vi "square_brackets_beside_vertical_bar_solution.vi"(8 "error in (no error)":errorcluster, 11 "Instrument Command In":string) -> (0 "error out":errorcluster, 3 "Instrument Command Out":string)   [LabVIEW 2018]
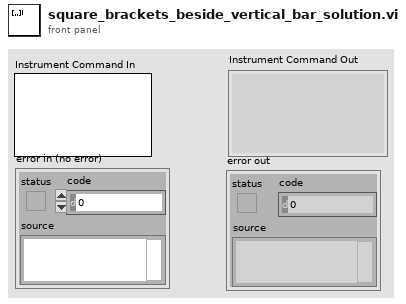
[diagram p1: front panel]
types:
  T1 = cluster{"Start Sting":string, "End String":string}
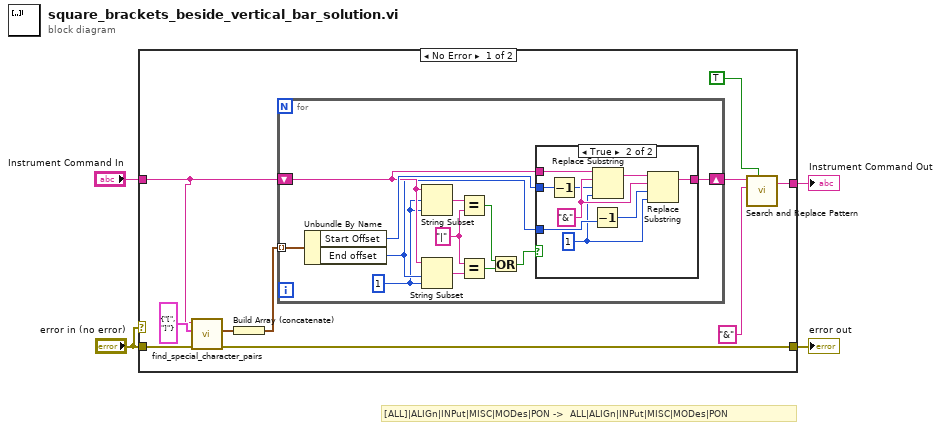
[diagram p0: block diagram]
diagram:
  # "[ALL]|ALIGn|INPut|MISC|MODes|PON ->  ALL|ALIGn|INPut|MISC|MODes|PON"
  n1 = case shown="No Error" "error in (no error)" {
    selector: "error in (no error)" -> [_ w38]
    tunnel: "Instrument Command In" -> [w5 w37]
    tunnel: "error in (no error)" -> [w9 _]
    tunnel: [w8 w38] -> w3
    tunnel: [w6 w37] -> w2
    frame No Error {
      n2 = call "find_special_character_pairs.vi"("error in (no error)"=w9, "String Pair"=T1 {"Start Sting"="[", "End String"="]"}, "Command String"=w5) -> ("error out"=w8:errorcluster, "Pair Offset"=w11:cluster{"Start Offset":i32, "End offset":i32}[])  [unwired: 7 out]
      n3 = Build Array (concatenate)(w11) -> (w10:cluster{"Start Offset":i32, "End offset":i32}[])
      n4 = for {
        shift-right: [w18] -> w13
        shift-left: w5 -> [w19]
        tunnel: w10 -> [w15] mode=indexing
        w24 = "|"
        w16 = 1
        n5 = Unbundle By Name(w15) -> ("Start Offset"=w20:i32, "End offset"=w17:i32)
        n6 = String Subset(string=w19, offset (0)=w16, length (rest)=w16) -> (substring=w26:string)
        n7 = String Subset(string=w19, offset (0)=w17, length (rest)=w16) -> (substring=w25:string)
        n8 = Equal?(x=w26, y=w24) -> (x = y?=w23:bool)
        n9 = Equal?(x=w24, y=w25) -> (x = y?=w22:bool)
        n10 = Or(x=w23, y=w22) -> (x .or. y?=w21:bool)
        n11 = case shown="True" w21 {
          tunnel: w20 -> [_ w36]
          tunnel: w19 -> [w27 w35]
          tunnel: w17 -> [_ w32]
          tunnel: [w27 w30] -> w18
          frame False {
          }
          frame True {
            w33 = "&" ("substring (\"\")")
            w31 = 1 ("length (len. of substring)")
            n12 = Decrement(x=w36) -> (x-1=w28:i32)
            n13 = Decrement(x=w32) -> (x-1=w29:i32)
            n14 = Replace Substring(2:w31, 3:w28, 4:w33, 5:w35) -> (1:w34:string)  [unwired: 1 out]
            n15 = Replace Substring(2:w31, 3:w29, 4:w33, 5:w34) -> (1:w30:string)  [unwired: 1 out]
          }
        }
      }
      n16 = call <vilib>:"Search and Replace Pattern.vi"("string"=w13, "regular expression (\"\")"="&" ("regular expression (\"\")"), "replace all? (F)"=TRUE) -> ("result string"=w6:string)  [unwired: 1 in, 2 out]
    }
    frame Error {
    }
  }
  "error out" <- w3
  "Instrument Command Out" <- w2
